vi "TB Global 1.vi"() -> ()   [LabVIEW 2019, in "Test Bench Tools.lvlib"]
uses:
  Test Bench Tools.lvlib
panel:
  in  "writer endpoint 4":refnum<k21>
  in  "writer endpoint 3":refnum<k21>
  in  "writer endpoint 2":refnum<k21>
  in  "writer endpoint 1":refnum<k21>
  in  "size(s)":i32
  in  "Sequence writer endpoint 4":refnum<k21>
  in  "Sequence writer endpoint 3":refnum<k21>
  in  "Sequence writer endpoint 2":refnum<k21>
  in  "Sequence writer endpoint 1":refnum<k21>
  in  "Terminate writer endpoint 4":refnum<k21>
  in  "Terminate writer endpoint 3":refnum<k21>
  in  "Terminate writer endpoint 2":refnum<k21>
  in  "Terminate writer endpoint 1":refnum<k21>
  in  "Exit writer endpoint 4":refnum<k21>
  in  "Exit writer endpoint 3":refnum<k21>
  in  "Exit writer endpoint 2":refnum<k21>
  in  "Exit writer endpoint 1":refnum<k21>
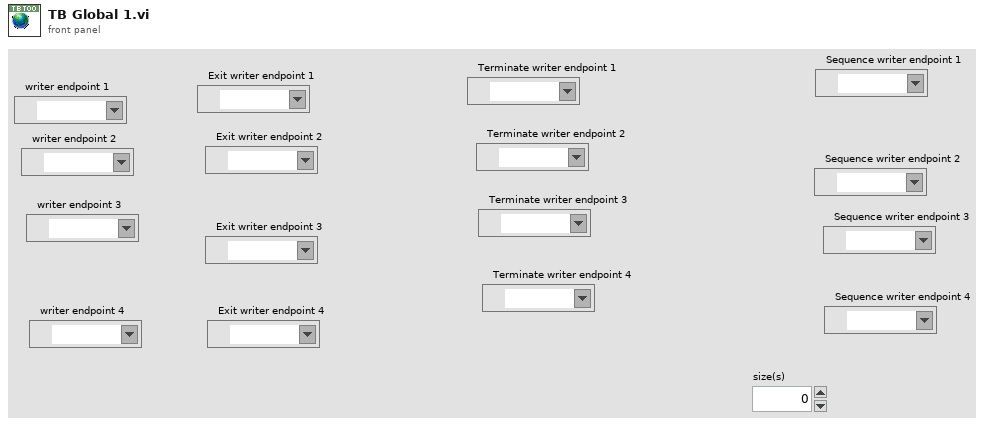
[diagram p1: front panel]
diagram:
